vi "Read Overlay.vi"(8 "error in (no error)":errorcluster, 11 "Analyze BaseClass in":refnum<class "Analyze BaseClass.lvclass">) -> (0 "error out":errorcluster, 2 "Overlay?":bool, 3 "Analyze BaseClass out":refnum<class "Analyze BaseClass.lvclass">)   [LabVIEW 2020, in "Analyze.lvlib" / "Analyze BaseClass.lvclass"]
uses:
  Analyze BaseClass.lvclass
  Analyze BaseClass.lvclass/Analyze BaseClass.ctl
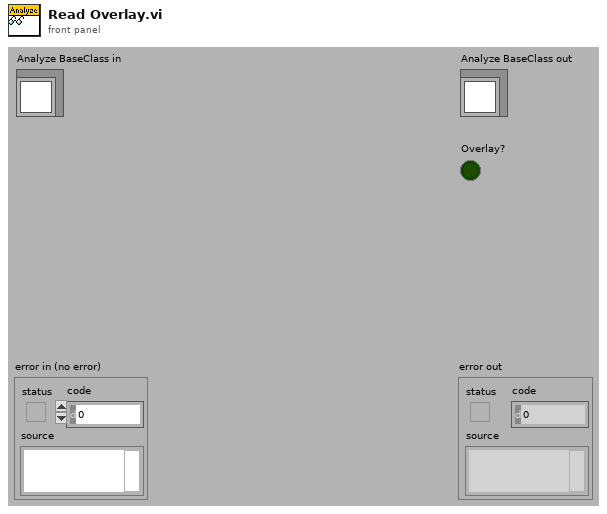
[diagram p1: front panel]
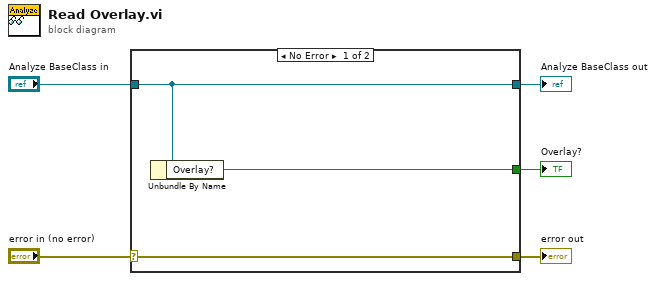
[diagram p0: block diagram]
diagram:
  n1 = case shown="No Error" "error in (no error)" {
    selector: "error in (no error)" -> [w8 w9]
    tunnel: [w8 w9] -> w4
    tunnel: [w7 w10] -> w2
    tunnel: "Analyze BaseClass in" -> [w7 w10]
    tunnel: [w6 _] -> w1
    frame No Error {
      n2 = Unbundle By Name(w7) -> ("Overlay?"=w6:bool)
    }
    frame Error {
    }
  }
  "error out" <- w4
  "Analyze BaseClass out" <- w2
  "Overlay?" <- w1
